vi "Write Base.vi"(8 "error in (no error)":errorcluster, 10 "Base":refnum<class "Base.lvclass">, 11 "Base Class Test In":refnum<class "Base Test.lvclass">) -> (0 "error out":errorcluster, 3 "Base Class Test Out":refnum<class "Base Test.lvclass">)   [LabVIEW 2020, in "Base Test.lvclass"]
uses:
  Base Test.lvclass
  Framework/Base/Base.lvclass
  Base Test.lvclass/Base Test.ctl
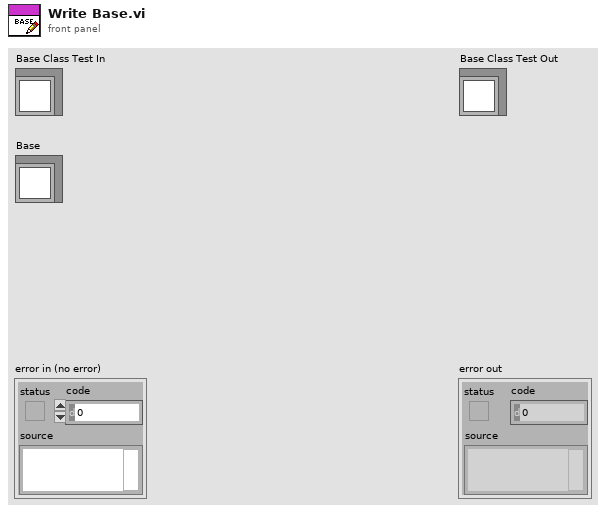
[diagram p1: front panel]
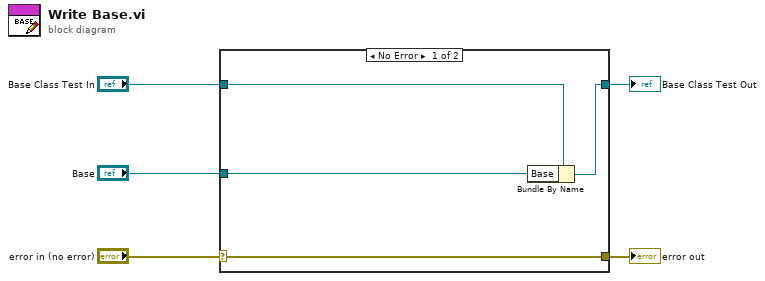
[diagram p0: block diagram]
diagram:
  n1 = case shown="No Error" "error in (no error)" {
    selector: "error in (no error)" -> [w9 w10]
    tunnel: [w9 w10] -> w4
    tunnel: [w7 w11] -> w2
    tunnel: "Base Class Test In" -> [w8 w11]
    tunnel: "Base" -> [w6 _]
    frame No Error {
      n2 = Bundle By Name(cluster=w8, "Base"=w6) -> (w7:refnum<class "Base Test.lvclass">)
    }
    frame Error {
    }
  }
  "error out" <- w4
  "Base Class Test Out" <- w2
